vi "SetActiveWindow.vi"(2 "error in (no error)":errorcluster, 3 "WindowHandle":T1) -> (0 "error out":errorcluster, 1 "Previous WindowHandle":T1)   [LabVIEW 2009]
doc: "Activates the Window referenced by \"WindowHandle\" and returns the handle of the previously activated window in \"Previous WindowHandle\".\nIf \"ErrorIn\" is TRUE nothing happens and \"Previous WindowHandle\" returns \"Not a Refnum\"."
uses:
  USER32.DLL
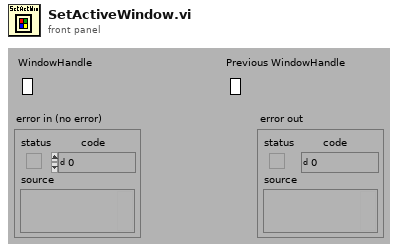
[diagram p1: front panel]
types:
  T1 = typedef "WindowHandle" = refnum<k1>
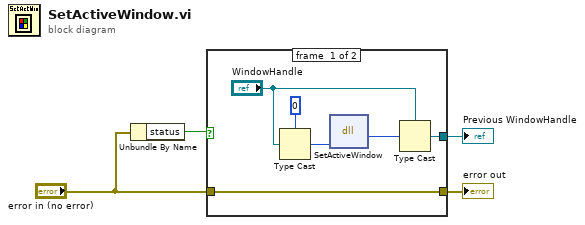
[diagram p0: block diagram]
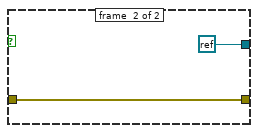
[diagram p2: hidden frame]
diagram:
  n1 = Unbundle By Name("error in (no error)") -> ("status"=w1:bool)
  n2 = case shown="True" w1 {
    tunnel: [w8 refnum<k0> refnum] -> w4
    tunnel: "error in (no error)" -> [w5 w12]
    tunnel: [w5 w12] -> w3
    frame #0 {
      n3 = Type Cast(type=u32 0, x="WindowHandle") -> (*(type *) &x=w10:u32)
      n4 = dll-call lib="USER32.DLL" fn="SetActiveWindow"("wHnd"=w10) -> (w7:u32)  [unwired: 4 in, 2 out]
      n5 = Type Cast(type="WindowHandle", x=w7) -> (*(type *) &x=w8:T1)
    }
    frame #1 {
    }
  }
  "Previous WindowHandle" <- w4
  "error out" <- w3
